vi "SwerveUnwrapGoalAngle.vi"(1 "Current Unwrapped Angle (deg) [-Inf,+Inf]":dbl, 2 "Flipped Goal Angle (deg) [-180, +180]":dbl) -> (0 "Absolute Azimuth Position (tics) [-Inf,+Inf]":dbl)   [LabVIEW 2020]
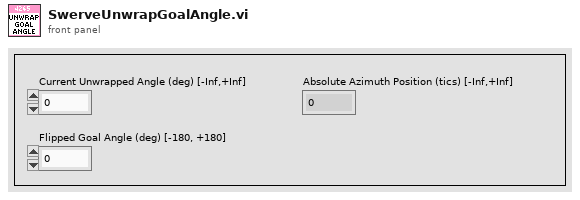
[diagram p1: front panel]
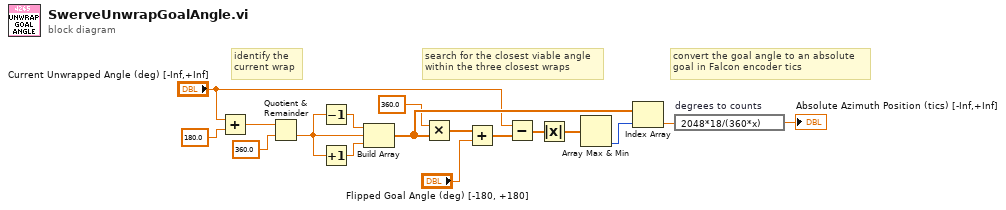
[diagram p0: block diagram]
diagram:
  # "convert the goal angle to an absolute\ngoal in Falcon encoder tics"
  # "search for the closest viable angle\nwithin the three closest wraps"
  # "identify the\ncurrent wrap"
  n1 = Add(x="Current Unwrapped Angle (deg) [-Inf,+Inf]", y=180.0) -> (x+y=w2:dbl)
  n2 = Quotient & Remainder(x=w2, y=360.0) -> (floor(x/y)=w6:dbl)  [unwired: 1 out]
  n3 = Decrement(x=w6) -> (x-1=w5:dbl)
  n4 = Increment(x=w6) -> (x+1=w7:dbl)
  n5 = Build Array(w5, w6, w7) -> (w15:dbl[])
  n6 = Multiply(x=360.0, y=w15) -> (x*y=w8:dbl[])
  n7 = Add(x=w8, y="Flipped Goal Angle (deg) [-180, +180]") -> (x+y=w10:dbl[])
  n8 = Subtract(x="Current Unwrapped Angle (deg) [-Inf,+Inf]", y=w10) -> (x-y=w12:dbl[])
  n9 = Absolute Value(x=w12) -> (abs(x)=w13:dbl[])
  n10 = Array Max & Min(array=w13) -> (min index (indices)=w14:i32)  [unwired: 3 out]
  n11 = Index Array(array=w15, index=w14) -> (element=w16:dbl)
  n12 = expression code="2048*18/(360*x)" "degrees to counts"(w16) -> (→"Absolute Azimuth Position (tics) [-Inf,+Inf]":dbl)
